vi "PV HiScroll Set value settings.vi"(8 "error in (no error)":errorcluster, 9 "PV HiScroll Set value settings - Cluster":T1={"Parameter"=enum."Setpoint in speed setting mode (707)", "Parameter\nread only<->describe"=FALSE, "Setpoint in speed setting mode [707]"=83.0, "Setpoint speed in standby operation [717]"=66.7, "Pressure 1 [hPa] (740)"=0, "Switch-on threshold (730)"=10.0, "Switch-off threshold (732)"=20.0, "Gas correction factor (742)"=1.0, "Unit adress (797)"=1} caption="Operating adjustment - Cluster" {"Switch-off threshold (732)" min=1.0 max=100.01 step=0.01 format="%.2f"; "Pressure 1 [hPa] (740)" min=0 max=2050 step=1; "Gas correction factor (742)" min=0.2 max=9.9 step=0.01 format="%.2f"; "Switch-on threshold (730)" min=0.01 max=30.01 step=0.01 format="%.2f"; "Unit adress (797)" min=1 max=255 step=1; "Setpoint speed in standby operation [717]" min=20.0 max=100.0 step=0.1 format="%.2f"; "Setpoint in speed setting mode [707]" min=20.0 max=100.0 step=0.1 format="%.2f"}, 10 "Adress of unit":u16=1 min=1 max=999 step=1, 11 "VISA session":refnum<visa-resource-name>) -> (0 "error out":errorcluster, 2 "response (data)":string, 3 "dup VISA session":refnum<visa-resource-name>)   [LabVIEW 2021, in "Pfeiffer Vacuum.lvlib"]
doc: "There are 7 parameters available, only one of which can be enabled at a time. \n\nSetpoint in speed setting mode (707)\nPower consumption limitation (708)\nSetpoint speed in standby operation (717)\nName sensor 1 (739)\nPressure 1 (740)\nGas correction factor 1 (742)\nRS-485 interface address (797)\n\nNote: The controls right of this one will set the appropriate values for the selected parameter. Any settings for an parameter that is not selected will be ignored. If a value is out of range, it will be changed to either the upper or the lower limit of the range."
uses:
  <instrlib>/Pfeiffer Vacuum/Pfeiffer Vacuum.lvlib
  <instrlib>/Pfeiffer Vacuum/Public/HiScroll/PV HiScroll Set value settings - Cluster.ctl
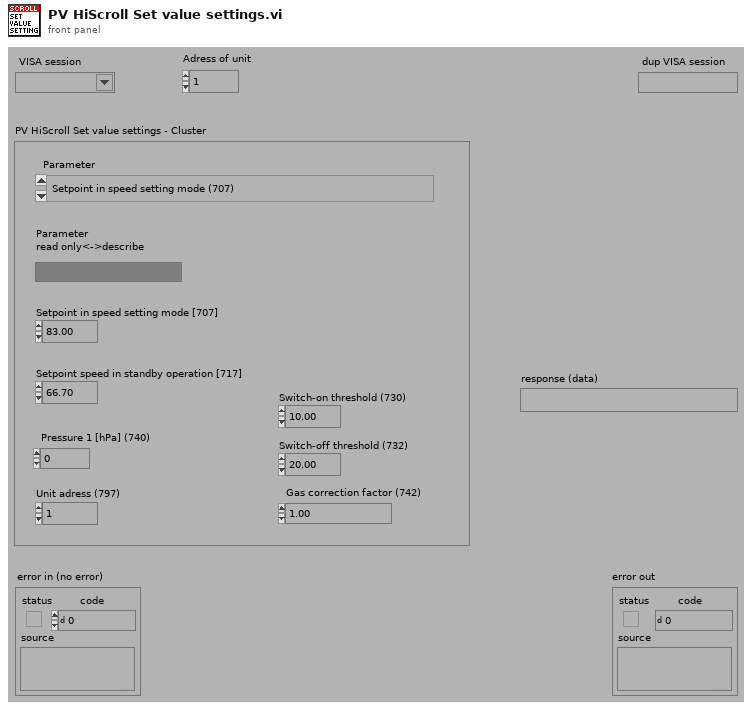
[diagram p1: front panel]
types:
  T1 = typedef "Pfeiffer Vacuum.lvlib/PV HiScroll Set value settings - Cluster.ctl" = cluster{"Parameter":enum16{"Setpoint in speed setting mode (707)", "Setpoint speed in standby operation (717)", "Switch-on threshold (Auto-Standby) [730]", "Switch-off threshold (Auto-Standby) [732]", "Name sensor 1 (739)", "Pressure 1 (740)", "Gas correction factor 1 (742)", "RS-485 interface address (797)"}, "Parameter\nread only<->describe":bool, "Setpoint in speed setting mode [707]":dbl, "Setpoint speed in standby operation [717]":dbl, "Pressure 1 [hPa] (740)":i16, "Switch-on threshold (730)":dbl, "Switch-off threshold (732)":dbl, "Gas correction factor (742)":sgl, "Unit adress (797)":i16}
  T2 = enum16{"Setpoint in speed setting mode (707)", "Setpoint speed in standby operation (717)", "Switch-on threshold (Auto-Standby) [730]", "Switch-off threshold (Auto-Standby) [732]", "Name sensor 1 (739)", "Pressure 1 (740)", "Gas correction factor 1 (742)", "RS-485 interface address (797)"}
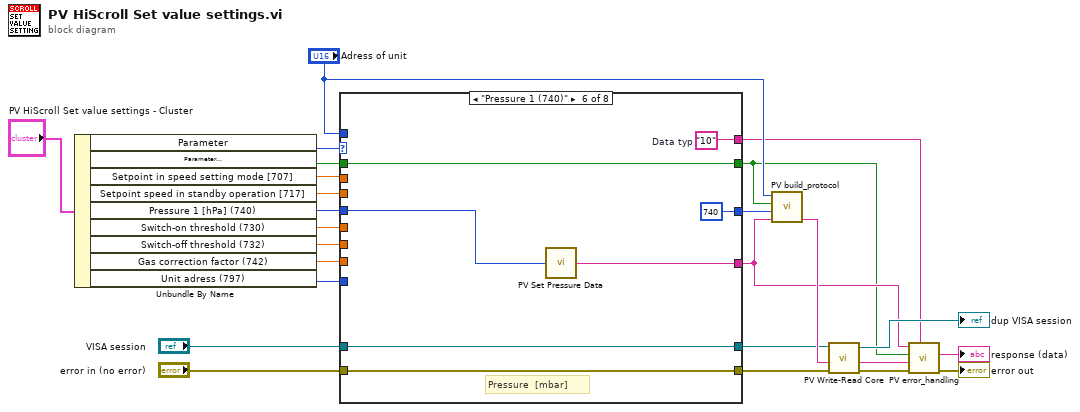
[diagram p0: block diagram]
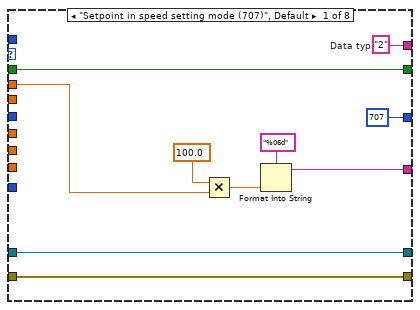
[diagram p2: hidden frame]
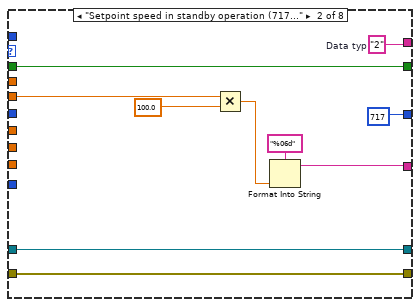
[diagram p3: hidden frame]
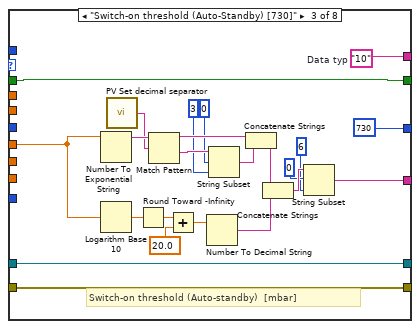
[diagram p4: hidden frame]
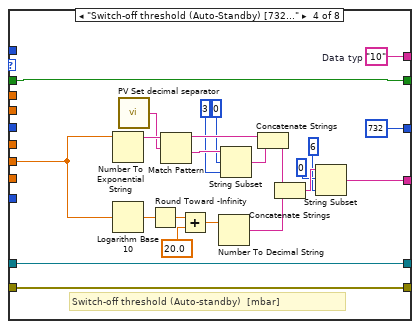
[diagram p5: hidden frame]
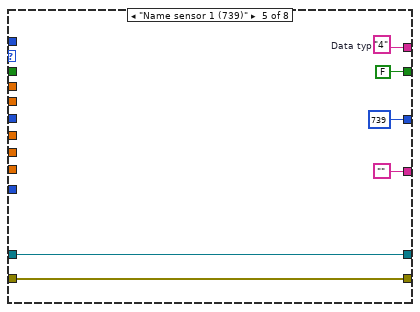
[diagram p6: hidden frame]
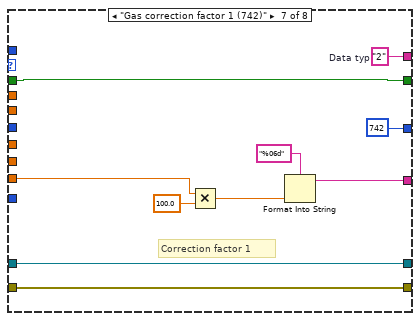
[diagram p7: hidden frame]
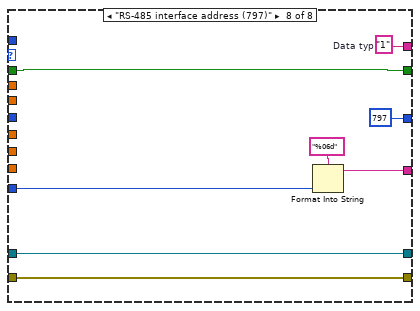
[diagram p8: hidden frame]
diagram:
  n1 = Unbundle By Name("PV HiScroll Set value settings - Cluster") -> ("Parameter"=w24:T2, "Parameter\nread only<->describe"=w23:bool, "Setpoint in speed setting mode [707]"=w8:dbl, "Setpoint speed in standby operation [717]"=w6:dbl, "Pressure 1 [hPa] (740)"=w3:i16, "Switch-on threshold (730)"=w5:dbl, "Switch-off threshold (732)"=w4:dbl, "Gas correction factor (742)"=w2:sgl, "Unit adress (797)"=w1:i16)
  n2 = case shown="\"Pressure 1 (740)\"" w24 {
    tunnel: [u16 707 ("Parameter-number") u16 717 ("Parameter-number") u16 730 ("Parameter-number") u16 732 ("Parameter-number") u16 739 ("Parameter-number") u16 740 ("Parameter-number") u16 742 ("Parameter-number") u16 797 ("Parameter-number")] -> w25
    tunnel: [w27 w37 w47 w70 "" w98 w110 w116] -> w13
    tunnel: [w30 w41 w65 w88 FALSE ("Parameter\nread only<->describe") w101 w109 w119] -> w11
    tunnel: w23 -> [w30 w41 w65 w88 _ w101 w109 w119]
    tunnel: w8 -> [w26 _ _ _ _ _ _ _]
    tunnel: w6 -> [_ w36 _ _ _ _ _ _]
    tunnel: [w29 w43 w64 w87 w94 w100 w108 w118] -> w12
    tunnel: "VISA session" -> [w35 w45 w68 w91 w97 w104 w114 w122]
    tunnel: [w35 w45 w68 w91 w97 w104 w114 w122] -> w18
    tunnel: "Adress of unit" -> [_ _ _ _ _ _ _ _]
    tunnel: "error in (no error)" -> [w34 w44 w67 w90 w96 w103 w113 w121]
    tunnel: [w34 w44 w67 w90 w96 w103 w113 w121] -> w17
    tunnel: w5 -> [_ _ w46 _ _ _ _ _]
    tunnel: w4 -> [_ _ _ w69 _ _ _ _]
    tunnel: w3 -> [_ _ _ _ _ w99 _ _]
    tunnel: w2 -> [_ _ _ _ _ _ w105 _]
    tunnel: w1 -> [_ _ _ _ _ _ _ w115]
    frame "Setpoint in speed setting mode (707)", Default {
      w29 = "2"  # Data typ
      n3 = Multiply(x=100.0, y=w26) -> (x*y=w32:dbl)
      n4 = Format Into String(format string="%06d" ("Format-String"), w32) -> (resulting string=w27:string)  [unwired: 2 in, 1 out]
    }
    frame "Setpoint speed in standby operation (717)" {
      w43 = "2"  # Data typ
      n5 = Multiply(x=w36, y=100.0) -> (x*y=w40:dbl)
      n6 = Format Into String(format string="%06d" ("Format-String"), w40) -> (resulting string=w37:string)  [unwired: 2 in, 1 out]
    }
    frame "Switch-on threshold (Auto-Standby) [730]" {
      w64 = "10"  # Data typ
      # "Switch-on threshold (Auto-standby)  [mbar]"
      n7 = Number To Exponential String(number=w46) -> (E-format string=w60:string)  [unwired: 3 in]
      n8 = Logarithm Base 10(1:w46) -> (0:w63:dbl)
      n9 = call <instrlib>:"PV Set decimal separator.vi"() -> ("decimal separator"=w48:string)
      n10 = Round Toward -Infinity(1:w63) -> (0:w62:dbl)
      n11 = Match Pattern(string=w60, regular expression=w48) -> (before substring=w61:string, after substring=w59:string)  [unwired: 1 in, 2 out]
      n12 = Add(x=w62, y=20.0) -> (x+y=w55:dbl)
      n13 = Number To Decimal String(number=w55) -> (decimal integer string=w52:string)  [unwired: 1 in]
      n14 = String Subset(string=w59, offset (0)=0 ("Offset (0)"), length (rest)=3 ("Länge")) -> (substring=w56:string)
      n15 = Concatenate Strings(w61, w56) -> (w53:string)
      n16 = Concatenate Strings(w53, w52) -> (w51:string)
      n17 = String Subset(string=w51, offset (0)=0 ("Offset (0)"), length (rest)=6 ("Länge")) -> (substring=w47:string)
    }
    frame "Switch-off threshold (Auto-Standby) [732]" {
      w87 = "10"  # Data typ
      # "Switch-off threshold (Auto-standby)  [mbar]"
      n18 = Number To Exponential String(number=w69) -> (E-format string=w83:string)  [unwired: 3 in]
      n19 = Logarithm Base 10(1:w69) -> (0:w86:dbl)
      n20 = call <instrlib>:"PV Set decimal separator.vi"() -> ("decimal separator"=w71:string)
      n21 = Round Toward -Infinity(1:w86) -> (0:w85:dbl)
      n22 = Match Pattern(string=w83, regular expression=w71) -> (before substring=w84:string, after substring=w82:string)  [unwired: 1 in, 2 out]
      n23 = Add(x=w85, y=20.0) -> (x+y=w78:dbl)
      n24 = Number To Decimal String(number=w78) -> (decimal integer string=w75:string)  [unwired: 1 in]
      n25 = String Subset(string=w82, offset (0)=0 ("Offset (0)"), length (rest)=3 ("Länge")) -> (substring=w79:string)
      n26 = Concatenate Strings(w84, w79) -> (w76:string)
      n27 = Concatenate Strings(w76, w75) -> (w74:string)
      n28 = String Subset(string=w74, offset (0)=0 ("Offset (0)"), length (rest)=6 ("Länge")) -> (substring=w70:string)
    }
    frame "Name sensor 1 (739)" {
      w94 = "4"  # Data typ
    }
    frame "Pressure 1 (740)" {
      w100 = "10"  # Data typ
      # "Pressure  [mbar]"
      n29 = call <instrlib>:"PV Set Pressure Data.vi"("Pressure (mbar)\n0 ==> ur (<1,0e-4mbar)\n1 - 2050 mbar"=w99) -> ("Output"=w98:string)
    }
    frame "Gas correction factor 1 (742)" {
      w108 = "2"  # Data typ
      # "Correction factor 1"
      n30 = Multiply(x=w105, y=100.0) -> (x*y=w106:dbl)
      n31 = Format Into String(format string="%06d" ("Format-String"), w106) -> (resulting string=w110:string)  [unwired: 2 in, 1 out]
    }
    frame "RS-485 interface address (797)" {
      w118 = "1"  # Data typ
      n32 = Format Into String(format string="%06d" ("Format-String"), w115) -> (resulting string=w116:string)  [unwired: 2 in, 1 out]
    }
  }
  n33 = call <instrlib>:"PV build_protocol.vi"("Data"=w13, "Parameter-number"=w25, "parameter\nread<->describe"=w11, "Adress"="Adress of unit") -> ("output"=w19:string)  [unwired: 3 in]
  n34 = call <instrlib>:"PV Write-Read Core.vi"("error in"=w17, "Write data in"=w19, "VISA session"=w18) -> ("error out"=w15:errorcluster, "response (data) out"=w16:string, "dup VISA session"=→"dup VISA session":refnum<visa-resource-name>)  [unwired: 2 in]
  n35 = call <instrlib>:"PV error_handling.vi"("Data Typ in"=w12, "error in"=w15, "response (data) in"=w16, "Parameter\nread only<->describe"=w11, "data in"=w13) -> ("error out"=→"error out":errorcluster, "Data out"=→"response (data)":string)  [unwired: 4 in, 1 out]
